vi "TDS RF Signal Output Power.vi"(8 "error in (no error)":errorcluster, 9 "Power":dbl, 10 "Signal InstConfig":string, 11 "Address":string) -> (0 "error out":errorcluster)   [LabVIEW 2025, in "Interface Functions.lvlib"]
uses:
  Interface Functions.lvlib
panel:
  out "read buffer":string
  # "RF Signal Output Power"
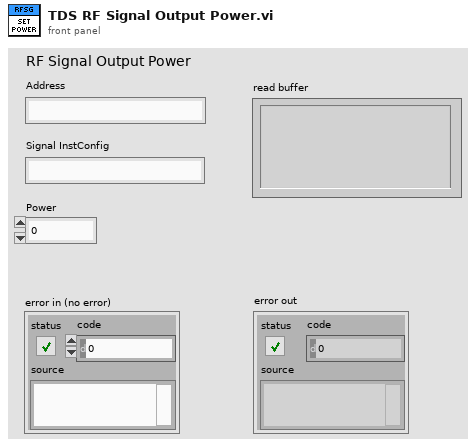
[diagram p1: front panel]
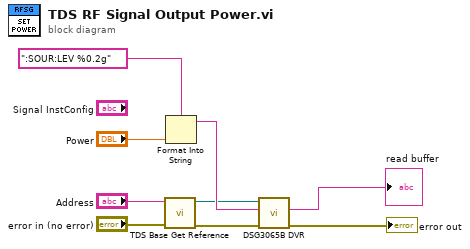
[diagram p0: block diagram]
diagram:
  n1 = call "TDS Base Get Reference.vi"("error in (no error)"="error in (no error)", "Address"="Address") -> ("error out"=w2:errorcluster, "Reference"=w1:refnum<visa-resource-name>)  [unwired: 8 in]
  n2 = Format Into String(format string=":SOUR:LEV %0.2g", "Power") -> (resulting string=w7:string)  [unwired: 2 in, 1 out]
  n3 = call "DSG3065B DVR.vi"("error in (no error)"=w2, "write buffer"=w7, "VISA resource name"=w1) -> ("error out"=→"error out":errorcluster, "read buffer"=→"read buffer":string)  [unwired: 7 in]
